vi "CheckNodeName.vi"(3 "node":string) -> (0 "name":string, 1 "Node":cluster{"name":string, "Port":u16})   [LabVIEW 2012]
uses:
  <userlib>/ROSforLV/ROS/Code/_ROSDefinition.vi
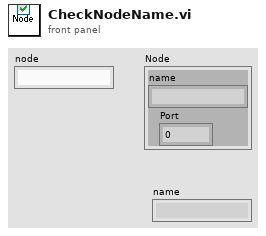
[diagram p1: front panel]
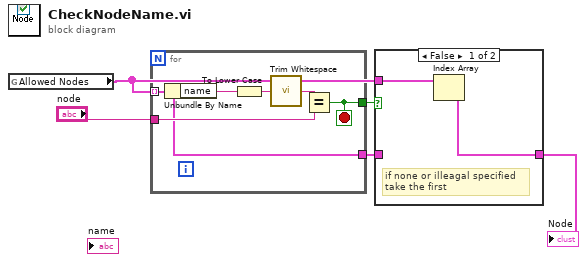
[diagram p0: block diagram]
diagram:
  n1 = global read "_ROSDefinition.vi" "Allowed Nodes"() -> (w4:cluster{"name":string, "Port":u16}[])
  n2 = for {
    tunnel: "node" -> [w9]
    tunnel: [w8] -> w2
    tunnel: [w7] -> w3
    tunnel: w4 -> [w7] mode=indexing
    stop <- w8 stop-if-true
    n3 = Unbundle By Name(w7) -> ("name"=w6:string)
    n4 = To Lower Case(string=w6) -> (all lower case string=w11:string)
    n5 = call <vilib>:"Trim Whitespace.vi"("string"=w11) -> ("trimmed string"=w10:string)  [unwired: 1 in]
    n6 = Equal?(x=w10, y=w9) -> (x = y?=w8:bool)
  }
  n7 = case shown="False" w2 {
    tunnel: [w12 w14] -> w5
    tunnel: w3 -> [_ w14]
    tunnel: w4 -> [w13 _]
    frame False {
      # "if none or illeagal specified\ntake the first"
      n8 = Index Array(array=w13) -> (element=w12:cluster{"name":string, "Port":u16})  [unwired: 1 in]
    }
    frame True {
    }
  }
  "Node" <- w5
